vi "test Create and Look Into Rx Execution Unit Map_RandomLabelsPerChannel_SDI_Disabled.vi"(8 "error in":errorcluster, 11 "TestCase in":refnum<class "Engine.lvclass">) -> (0 "error out":errorcluster, 3 "TestCase out":refnum<class "Engine.lvclass">)   [LabVIEW 2021, in "Engine.lvclass"]
uses:
  Engine.lvclass
  Shared/Parameter Definition.ctl
  <vilib>/NI/NI VeriStand Encoding and Decoding/Encoding.ctl
  Shared/RT Hardware Channel Settings.ctl
  Shared/RT Label Settings.ctl
  Shared/Label.ctl
  Shared/RT Parameters.ctl
  <vilib>/NI VeriStand/Custom Device API/Custom Device Item Ref.ctl
  Shared/Transfer Type.ctl
  <vilib>/NI VeriStand/Custom Device API/Data Reference.ctl
  <vilib>/numeric/Random Number (Range) U64.vi
  <vilib>/numeric/sub_Random U32.vi
  <vilib>/addons/_JKI Toolkits/VI Tester/TestCase.llb/TestCase.lvclass
  Engine/Custom Device/Custom Device.lvlib
  <vilib>/NI VeriStand/Custom Device API/Custom Device API.lvlib
  <vilib>/NI/NI VeriStand Encoding and Decoding/Encoding and Decoding.lvlib
  C:/Program Files/National Instruments/LabVIEW 2021/vi.lib/addons/_JKI Toolkits/VI Tester/TestCase.llb/TestCase.lvclass
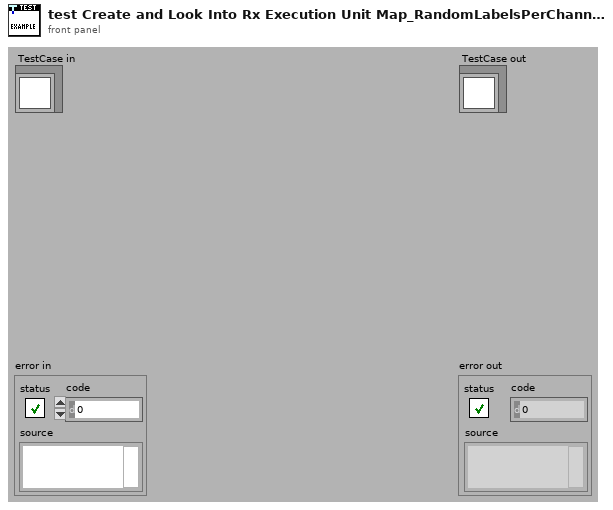
[diagram p1: front panel]
types:
  T1 = typedef "Parameter Definition.ctl" = cluster{"start index":i32, "size":i32, "encoding":T2, "signed":bool, "scale multiplier":dbl, "scale offset":dbl}
  T2 = typedef "Encoding and Decoding.lvlib/Encoding.ctl" = enum16{"BNR", "BCD", "Discrete"}
  T3 = typedef "RT Hardware Channel Settings.ctl" = cluster{"channel #":u16, "channel handle":u64, "labels settings for RT":T4[]}
  T4 = typedef "RT Label Settings.ctl" = cluster{"Name":string, "xmlName":string, "label":T5, "transfer period":u32, "SDI_Enabled":bool, "SDI":u8, "parameter driver data":T6, "transfer type":T8, "has timestamp?":bool, "Label Disable/Trigger Channel Reference":T7, "Message Handle":u64, "Initialized?":bool, "Word Initial Raw Value":u32, "Label Timestamp Channel Data Reference":T9, "disabled":bool}
  T5 = typedef "Label.ctl" = u8
  T6 = typedef "RT Parameters.ctl" = cluster{"parameter definitions":T1[], "Tx parameter refs":T7[]}
  T7 = typedef "Custom Device API.lvlib/Custom Device Item Ref.ctl" = u64
  T8 = typedef "Transfer Type.ctl" = enum16{"Scheduled", "Acyclic", "Block", "Strobe"}
  T9 = typedef "Custom Device API.lvlib/Data Reference.ctl" = i32
  T10 = cluster{"channel index":i32, "label index":i32, "start index":i32, "parameters":i32, "timestamp index":i32}
  T11 = typedef "Map of Identifiers to Indexes.ctl" = map{u32, cluster{"channel index":i32, "label index":i32, "start index":i32, "parameters":i32, "timestamp index":i32}}
  T12 = cluster{"channel index":i32, "label index":i32, "start index":i32, "parameters":i32, "timestamp index":i32}[]
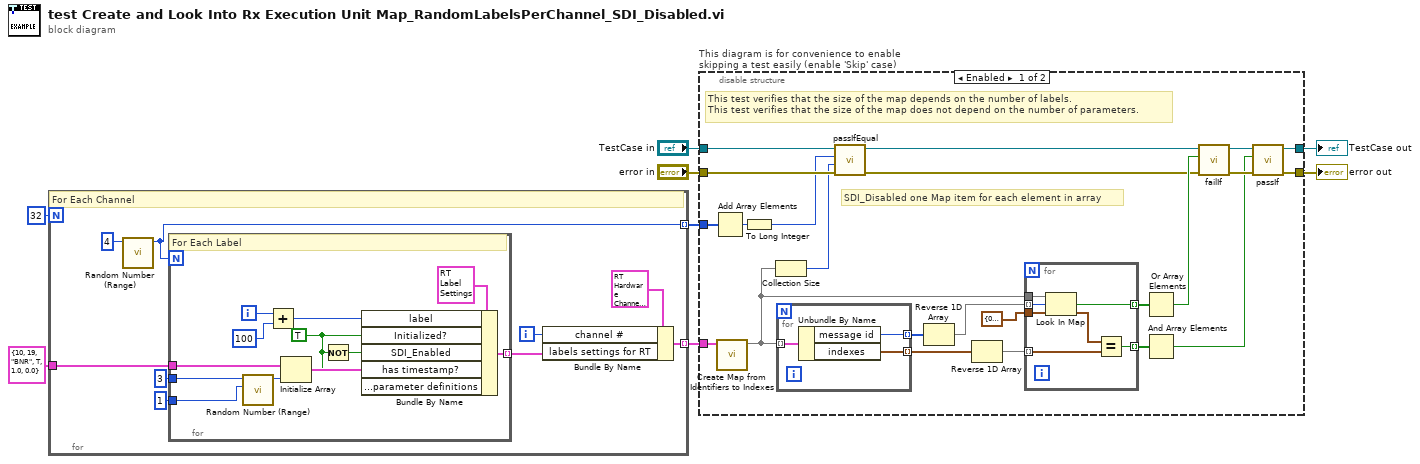
[diagram p0: block diagram]
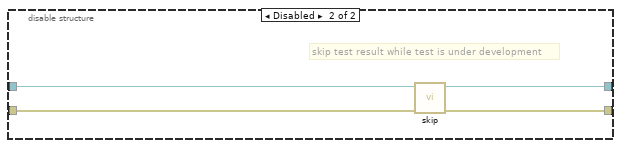
[diagram p2: hidden frame]
diagram:
  n1 = for {
    N: 32 -> [_]
    tunnel: T1 {"start index"=10, "size"=19, "encoding"=enum."BNR", "signed"=TRUE, "scale multiplier"=1.0, "scale offset"=0.0} ("parameter definition out") -> [w16]
    tunnel: [w12] -> w2 mode=indexing
    tunnel: [w11] -> w1 mode=indexing
    i -> [w13]
    # "For Each Channel"
    n2 = call-poly <vilib>:"Random Number (Range).vi"("upper bound (100)"=u64 4) -> ("number"=w11:u64)  [unwired: 10 in]
    n3 = for {
      N: w11 -> [_]
      tunnel: w16 -> [w25]
      tunnel: [w24] -> w15 mode=indexing
      tunnel: u64 3 ("upper bound (100)") -> [w21]
      tunnel: u64 1 ("upper bound (100)") -> [w20]
      i -> [w29]
      w19 = TRUE ("Initialized?")
      # "For Each Label"
      n4 = call-poly <vilib>:"Random Number (Range).vi"("lower bound (0)"=w20, "upper bound (100)"=w21) -> ("number"=w23:u64)  [unwired: 9 in]
      n5 = Add(x=w29, y=100) -> (x+y=w27:i32)
      n6 = Initialize Array(w25, w23) -> (w26:T1[])
      n7 = Not(x=w19) -> (.not. x?=w18:bool)
      n8 = Bundle By Name(cluster=T4 {"Name"="", "xmlName"="", "label"=0, "transfer period"=0, "SDI_Enabled"=FALSE, "SDI"=0, "parameter driver data"={"parameter definitions"=[], "Tx parameter refs"=[]}, "transfer type"=enum."Scheduled", "has timestamp?"=FALSE, "Label Disable/Trigger Channel Reference"=0, "Message Handle"=0, "Initialized?"=FALSE, "Word Initial Raw Value"=0, "Label Timestamp Channel Data Reference"=0, "disabled"=FALSE} ("label settings for RT"), "label"=w27, "Initialized?"=w19, "SDI_Enabled"=w18, "has timestamp?"=w19, "parameter driver data.parameter definitions"=w26) -> (w24:T4)
    }
    n9 = Bundle By Name(cluster=T3 {"channel #"=1, "channel handle"=0, "labels settings for RT"=[{"Name"="", "xmlName"="", "label"=11, "transfer period"=0, "SDI_Enabled"=FALSE, "SDI"=0, "parameter driver data"={"parameter definitions"=[{"start index"=10, "size"=16, "encoding"=enum."BCD", "signed"=TRUE, "scale multiplier"=1.0, "scale offset"=0.0}], "Tx parameter refs"=[]}, "transfer type"=enum."Scheduled", "has timestamp?"=TRUE, "Label Disable/Trigger Channel Reference"=0, "Message Handle"=0, "Initialized?"=TRUE, "Word Initial Raw Value"=0, "Label Timestamp Channel Data Reference"=0, "disabled"=FALSE}, {"Name"="", "xmlName"="", "label"=55, "transfer period"=0, "SDI_Enabled"=FALSE, "SDI"=0, "parameter driver data"={"parameter definitions"=[{"start index"=15, "size"=11, "encoding"=enum."BNR", "signed"=FALSE, "scale multiplier"=0.0, "scale offset"=0.0}], "Tx parameter refs"=[]}, "transfer type"=enum."Scheduled", "has timestamp?"=FALSE, "Label Disable/Trigger Channel Reference"=0, "Message Handle"=0, "Initialized?"=TRUE, "Word Initial Raw Value"=0, "Label Timestamp Channel Data Reference"=0, "disabled"=FALSE}, {"Name"="", "xmlName"="", "label"=77, "transfer period"=0, "SDI_Enabled"=FALSE, "SDI"=0, "parameter driver data"={"parameter definitions"=[{"start index"=10, "size"=4, "encoding"=enum."BCD", "signed"=FALSE, "scale multiplier"=0.0, "scale offset"=0.0}, {"start index"=14, "size"=2, "encoding"=enum."BNR", "signed"=FALSE, "scale multiplier"=0.0, "scale offset"=0.0}, {"start index"=16, "size"=12, "encoding"=enum."BNR", "signed"=FALSE, "scale multiplier"=0.0, "scale offset"=0.0}], "Tx parameter refs"=[]}, "transfer type"=enum."Scheduled", "has timestamp?"=FALSE, "Label Disable/Trigger Channel Reference"=0, "Message Handle"=0, "Initialized?"=TRUE, "Word Initial Raw Value"=0, "Label Timestamp Channel Data Reference"=0, "disabled"=FALSE}]} ("RT hardware channel"), "channel #"=w13, "labels settings for RT"=w15) -> (w12:T3)
  }
  n10 = disable-structure "This diagram is for convenience to enable skipping a test easily (enable 'Skip' case)" shown="Enabled" {
    disable-tunnel: "TestCase in" -> [w35 w66]
    disable-tunnel: [w52 w64] -> w5
    disable-tunnel: [w51 w65] -> w7
    disable-tunnel: "error in" -> [w34 w63]
    disable-tunnel: w2 -> [w50 _]
    disable-tunnel: w1 -> [w31 _]
    frame Enabled {
      # "SDI_Disabled one Map item for each element in array"
      # "This test verifies that the size of the map depends on the number of labels.\nThis test verifies that the size of the map does not depend on the number of parameters."
      n11 = Add Array Elements(numeric array=w31) -> (sum=w32:u64)
      n12 = call "Create Map from Identifiers to Indexes.vi"("RT hardware channel data"=w50) -> ("map from identifiers to indexes"=w38:T11)  [unwired: 10 in]
      n13 = To Long Integer(number=w32) -> (32bit integer=w30:i32)
      n14 = Collection Size(1:w38) -> (0:w33:i32)
      n15 = for {
        tunnel: w38 -> [w62] mode=indexing
        tunnel: [w61] -> w49 mode=indexing
        tunnel: [w60] -> w48 mode=indexing
        n16 = Unbundle By Name(w62) -> ("message id"=w61:u32, "indexes"=w60:T10)
      }
      n17 = call-dynamic "passIfEqual.vi"("error in (no error)"=w34, "y"=w33, "x"=w30, "TestCase in"=w35) -> ("error out"=w36:errorcluster, "TestCase out"=w37:refnum<class "Engine.lvclass">)  [unwired: 6 in]
      n18 = Reverse 1D Array(array=w49) -> (reversed array=w47:u32[])
      n19 = Reverse 1D Array(array=w48) -> (reversed array=w41:T12)
      n20 = for {
        tunnel: w38 -> [w59]
        tunnel: w47 -> [w58] mode=indexing
        tunnel: T10 {"channel index"=0, "label index"=0, "start index"=0, "parameters"=0, "timestamp index"=0} ("default value") -> [w57]
        tunnel: [w56] -> w45 mode=indexing
        tunnel: w41 -> [w54] mode=indexing
        tunnel: [w53] -> w40 mode=indexing
        n21 = Look In Map(map=w59, key=w58, default value=w57) -> (key not found?=w56:bool, value=w55:T10)
        n22 = Equal?(x=w55, y=w54) -> (x = y?=w53:bool)
      }
      n23 = Or Array Elements(Boolean array=w45) -> (logical OR=w44:bool)
      n24 = And Array Elements(Boolean array=w40) -> (logical AND=w39:bool)
      n25 = call-dynamic "failIf.vi"("error in (no error)"=w36, "fail"=w44, "TestCase in"=w37) -> ("error out"=w42:errorcluster, "TestCase out"=w43:refnum<class "Engine.lvclass">)  [unwired: 7 in]
      n26 = call-dynamic "passIf.vi"("error in (no error)"=w42, "pass"=w39, "TestCase in"=w43) -> ("error out"=w51:errorcluster, "TestCase out"=w52:refnum<class "Engine.lvclass">)  [unwired: 7 in]
    }
    frame Disabled {
      # "skip test result while test is under development"
      n27 = call <vilib>:"skip.vi"("error in (no error)"=w63, "TestCase in"=w66) -> ("error out"=w65:errorcluster, "TestCase out"=w64:refnum<class "Engine.lvclass">)  [unwired: 8 in]
    }
  }
  "error out" <- w7
  "TestCase out" <- w5
